vi "Query - Int64 - Scalar.vi"(8 "error in":errorcluster, 10 "Query":string, 11 "Module ID":i32=-1) -> (0 "error out":errorcluster, 1 "Meta Data":variant, 2 "Return Data":i64, 4 "Field Names":string[](array[string]))   [LabVIEW 2014, in "DB_CONNECTOR.lvlib"]
uses:
  DB_CONNECTOR.lvlib
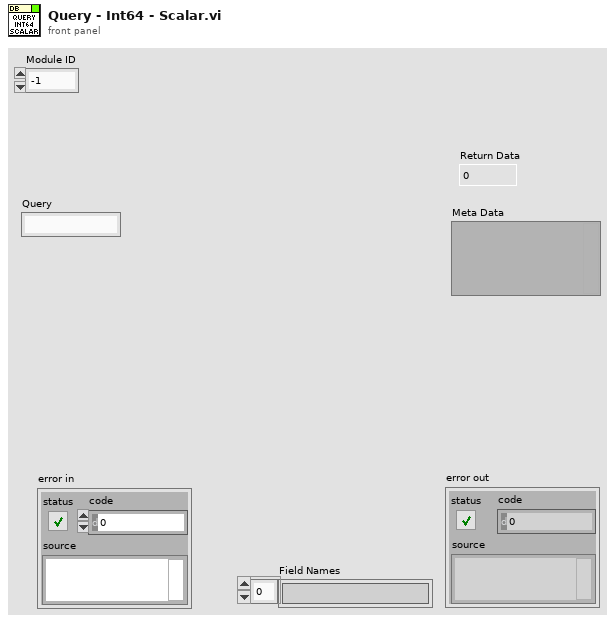
[diagram p1: front panel]
types:
  T1 = typedef "DB_CONNECTOR.lvlib/Query (Reply Payload)--cluster.ctl" = cluster{"Return Data":string[][], "Meta Data":variant, "Field Names":string[], "Query_error":errorcluster}
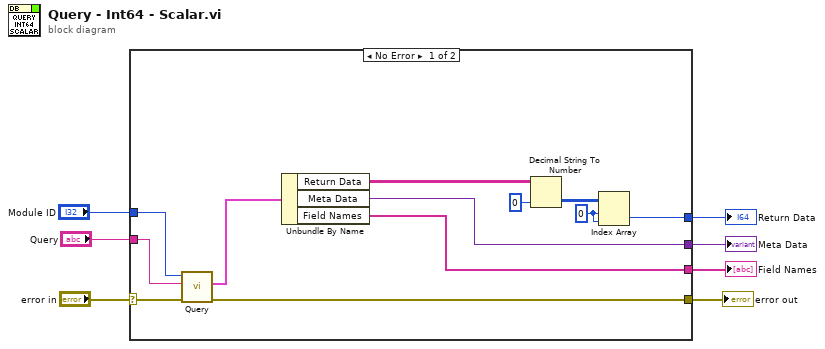
[diagram p0: block diagram]
diagram:
  n1 = case shown="No Error" "error in" {
    selector: "error in" -> [w19 w20]
    tunnel: [w10 w20] -> w6
    tunnel: "Query" -> [w11 _]
    tunnel: "Module ID" -> [w17 _]
    tunnel: [w9 _] -> w2
    tunnel: [w16 _] -> w3
    tunnel: [w8 _] -> w1
    frame No Error {
      w12 = 0 ("index (row)")
      n2 = call "Query.vi"("error in (no error)"=w19, "Query"=w11, "Module ID"=w17) -> ("error out"=w10:errorcluster, "Reply Payload"=w18:T1)  [unwired: 7 in]
      n3 = Unbundle By Name(w18) -> ("Return Data"=w15:string[][], "Meta Data"=w9:variant, "Field Names"=w8:string[])
      n4 = Decimal String To Number(string=w15, default (0L)=i64 0 ("default (0 I32)")) -> (number=w13:i64[][])  [unwired: 1 in, 1 out]
      n5 = Index Array(array=w13, index (row)=w12, index (col)=w12) -> (element=w16:i64)
    }
    frame Error {
    }
  }
  "error out" <- w6
  "Return Data" <- w3
  "Meta Data" <- w2
  "Field Names" <- w1
